vi "add.vi"(8 "error in (no error)":errorcluster, 10 "Input Frame":cdb[][](array[numeric]), 11 "Synchronizer in":refnum<class "Synchronizer.lvclass">) -> (0 "error out":errorcluster, 2 "Output Frame":cdb[][](array[numeric]), 3 "Synchronizer out":refnum<class "Synchronizer.lvclass">)   [LabVIEW 2012, in "Synchronizer.lvclass"]
uses:
  Synchronizer.lvclass
  Synchronizer.lvclass/Synchronizer.ctl
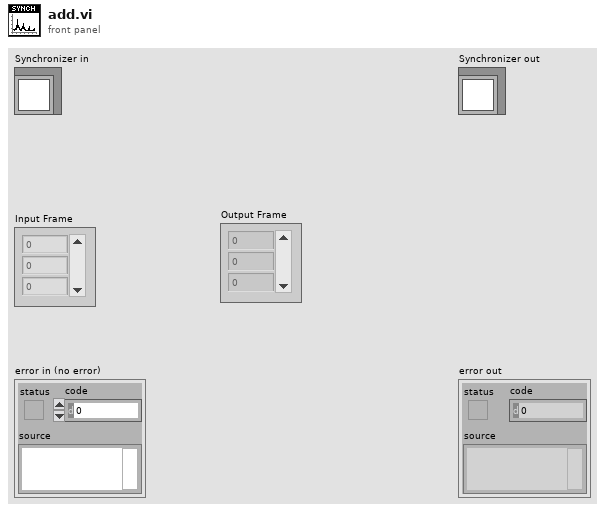
[diagram p1: front panel]
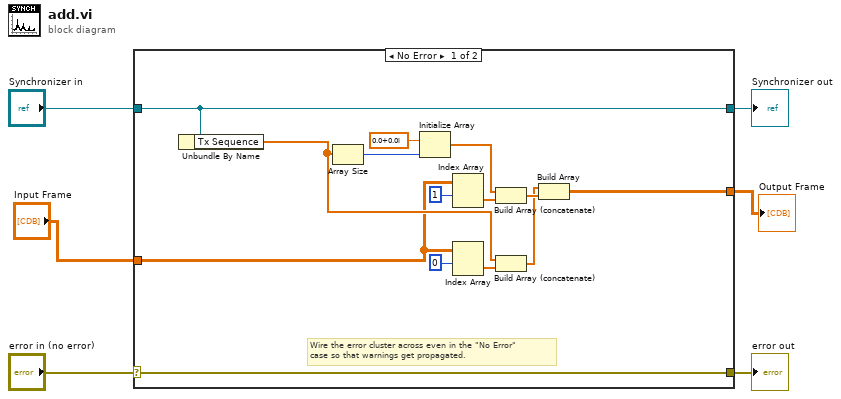
[diagram p0: block diagram]
diagram:
  n1 = case shown="No Error" "error in (no error)" {
    selector: "error in (no error)" -> [w20 w22]
    tunnel: [w20 w22] -> w5
    tunnel: [w9 w21] -> w3
    tunnel: "Synchronizer in" -> [w9 w21]
    tunnel: [w10 _] -> w1
    tunnel: "Input Frame" -> [w7 _]
    frame No Error {
      # "Wire the error cluster across even in the \"No Error\"\ncase so that warnings get propagated."
      n2 = Unbundle By Name(w9) -> ("Tx Sequence"=w8:cdb[])
      n3 = Array Size(array=w8) -> (size(s)=w12:i32)
      n4 = Initialize Array(cdb 0.0+0.0i ("element"), w12) -> (w18:cdb[])
      n5 = Index Array(array=w7, index (row)=1) -> (element=w17:cdb[])  [unwired: 1 in]
      n6 = Index Array(array=w7, index (row)=0) -> (element=w15:cdb[])  [unwired: 1 in]
      n7 = Build Array (concatenate)(w18, w17) -> (w19:cdb[])
      n8 = Build Array (concatenate)(w8, w15) -> (w11:cdb[])
      n9 = Build Array(w11, w19) -> (w10:cdb[][])
    }
    frame Error {
    }
  }
  "error out" <- w5
  "Synchronizer out" <- w3
  "Output Frame" <- w1
